vi "ResistanceToError.vi"(2 "Resistance / Ohms":dbl=25.0 format="%0.2f", 3 "Bridge settings":T1) -> (1 "Reading (-1 -> +1)":dbl)   [LabVIEW 2015]
uses:
  controls/BridgeSettings.ctl
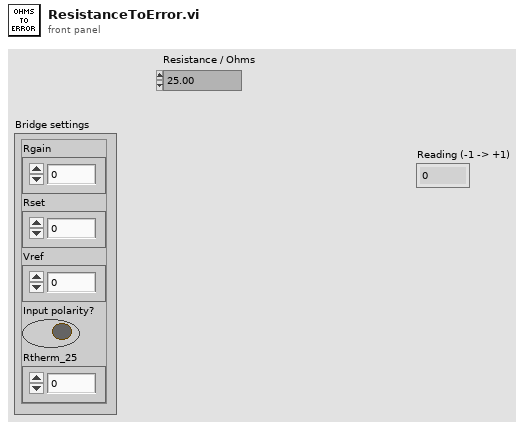
[diagram p1: front panel]
types:
  T1 = typedef "BridgeSettings.ctl" = cluster{"Rgain":dbl, "Rset":dbl, "Vref":dbl, "Input polarity?":bool, "Rtherm_25":dbl}
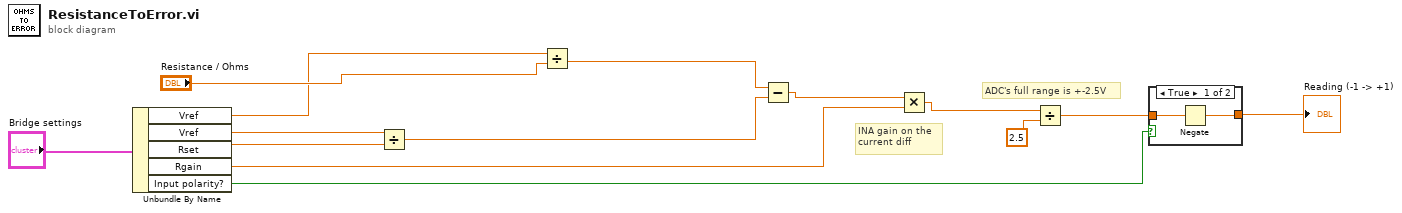
[diagram p0: block diagram]
diagram:
  # "INA gain on the\ncurrent diff"
  # "ADC's full range is +-2.5V"
  n1 = Unbundle By Name("Bridge settings") -> ("Vref"=w13:dbl, "Vref"=w12:dbl, "Rset"=w11:dbl, "Rgain"=w7:dbl, "Input polarity?"=w3:bool)
  n2 = Divide(x=w12, y=w11) -> (x/y=w9:dbl)
  n3 = Divide(x=w13, y="Resistance / Ohms") -> (x/y=w10:dbl)
  n4 = Subtract(x=w10, y=w9) -> (x-y=w8:dbl)
  n5 = Multiply(x=w8, y=w7) -> (x*y=w6:dbl)
  n6 = Divide(x=w6, y=2.5) -> (x/y=w4:dbl)
  n7 = case shown="True" w3 {
    tunnel: [w15 w17] -> w2
    tunnel: w4 -> [w16 w17]
    frame True {
      n8 = Negate(x=w16) -> (-x=w15:dbl)
    }
    frame False {
    }
  }
  "Reading (-1 -> +1)" <- w2
